vi "Funnel Edit.vi"() -> ()   [LabVIEW 2016]
uses:
  <userlib>/LevyLab/Relay Box/Type_defs/Resistor--enum.ctl
  Global Variables.vi
panel:
  in  "Set Resistance":T1=enum."1G ohm"
  in  "Index":i32=8
  in  "Direction":u16(ring) items=["Forward", "Backward"]
  in  "Enabled":bool=TRUE
  in  "Voltage Schedule":u16(ring) items=["Constant", "Ramp", "Fn. Generator", "Formula"]
  in  "Apply to All":bool
  in  "Smooth Segments":dbl=12.0
  in  "Speed Schedule":u16(ring) items=["Constant", "Ramp", "Fn. Generator", "Formula"]
  in  "Speed (µm/s)":dbl=8.0 min=1e-09
  in  "Voltage (V)":dbl=8.0
  in  "Speed Settings":bool
  in  "Voltage Settings":bool
  in  "Bottom Segs.":dbl=0.1
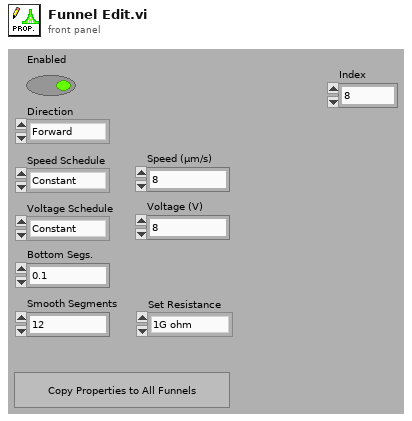
[diagram p1: front panel]
types:
  T1 = typedef "Resistor--enum.ctl" = enum16{"open", "discharge tip", "0 ohms", "100k ohm", "10M ohm", "1G ohm"}
  T2 = enum32{"invalid app kind", "Development System", "Run Time System", "Student Edition", "Embedded LabVIEW", "Evaluation", "Custom"}
  T3 = enum32{"Invalid", "Standard", "Closed", "Hidden", "Minimized", "Maximized"}
  T4 = typedef "Funnel Properties - cluster.ctl" = cluster{"Enabled":bool, "Direction":u16, "Smooth Segments":dbl, "Bottom Segs.":dbl, "Speed (um/s)":T5, "Voltage (V)":T5, "Set Resistance":T1}
  T5 = typedef "Voltage - cluster.ctl" = cluster{"Schedule":T6, "Value":dbl, "Start Value":dbl, "End Value":dbl, "Min Value":dbl, "Max Value":dbl, "Duty Cycle (%)":dbl, "Signal Type":T7, "Cycle Number":dbl, "Phase (degrees)":dbl, "formula":string, "formula length (nm)":dbl, "formula resolution (nm)":dbl}
  T6 = typedef "Schedule - enum.ctl" = enum16{"Constant", "Ramp", "Fn. Generator", "Formula"}
  T7 = typedef "Signal Type - enum.ctl" = enum16{"Sine Wave", "Triangle Wave", "Square Wave", "Sawtooth Wave"}
  T8 = cluster{"Core":cluster{"Current VI Reference":refnum<vi>, "Close Panel on Exit?":bool}}
  T9 = cluster{"Current VI Reference":refnum<vi>, "Close Panel on Exit?":bool}
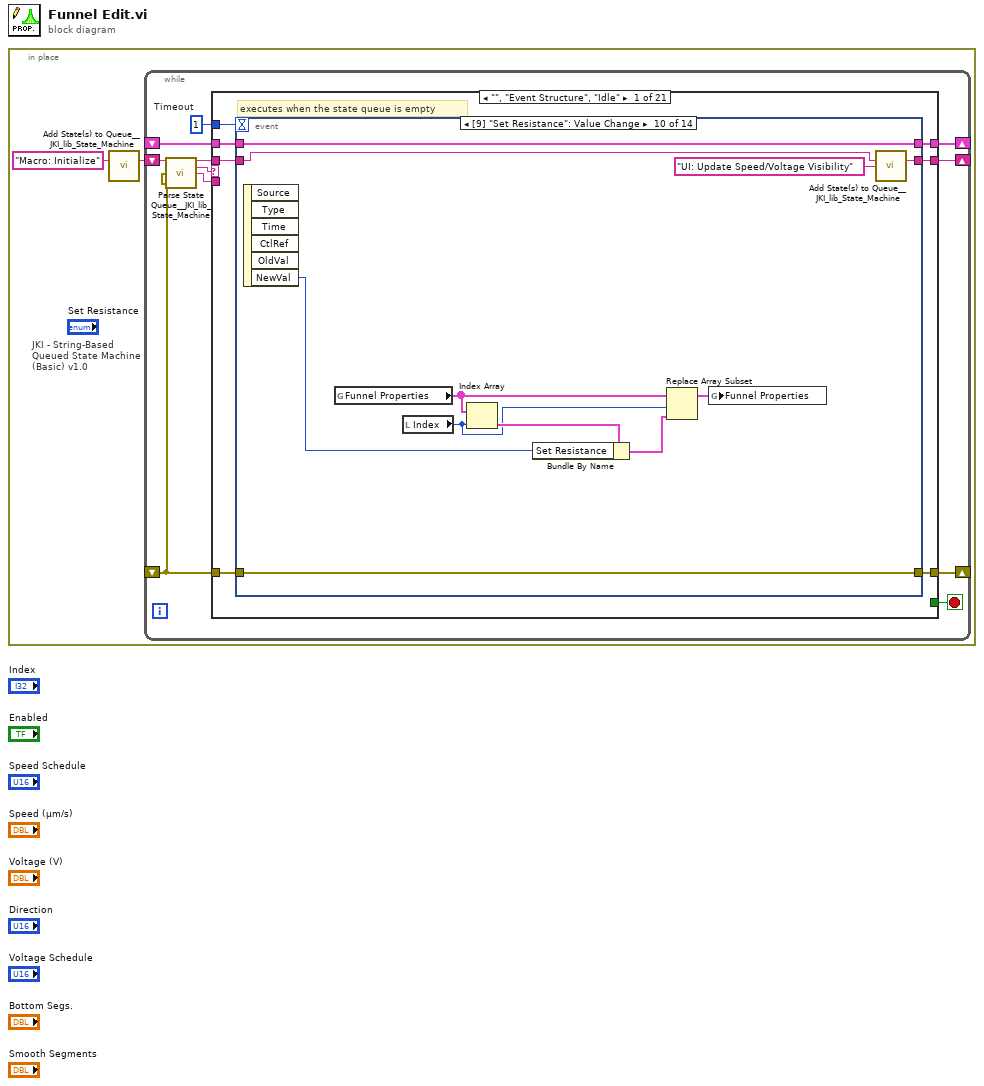
[diagram p0: block diagram]
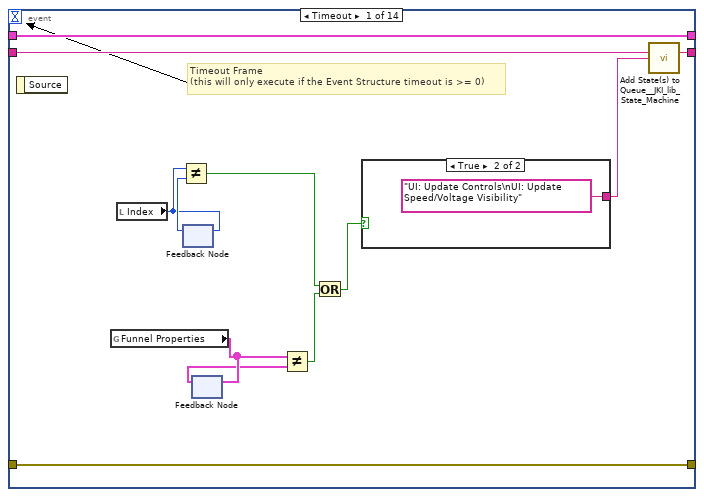
[diagram p2: hidden frame]
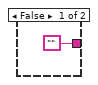
[diagram p3: hidden frame]
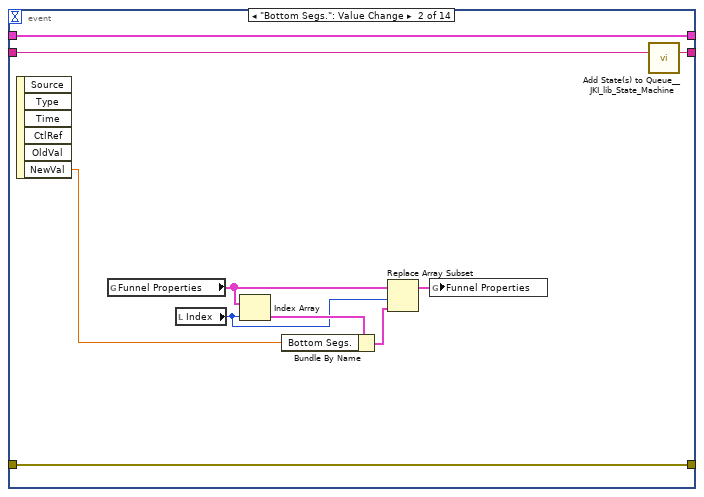
[diagram p4: hidden frame]
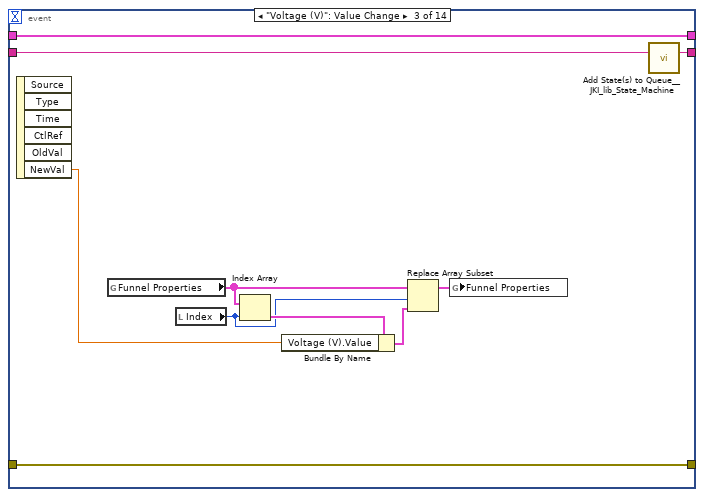
[diagram p5: hidden frame]
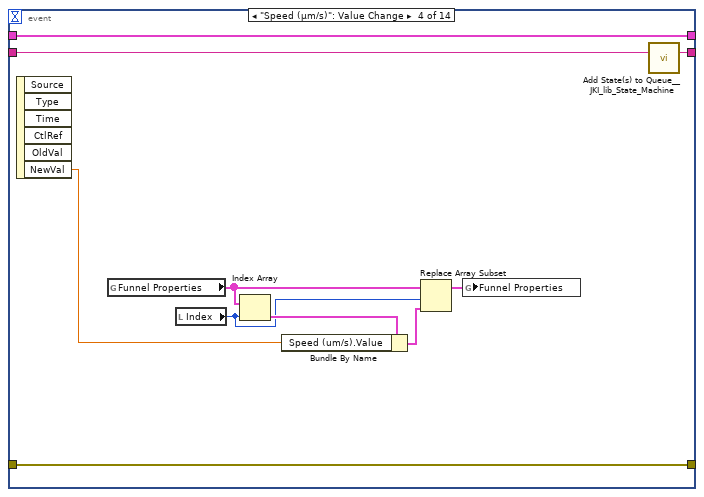
[diagram p6: hidden frame]
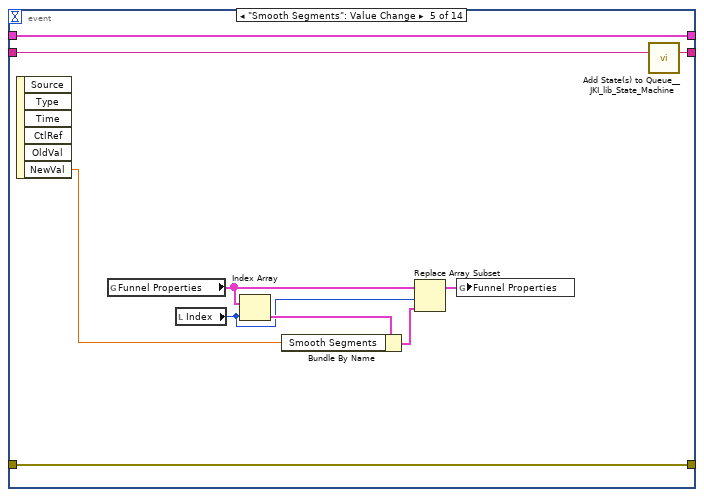
[diagram p7: hidden frame]
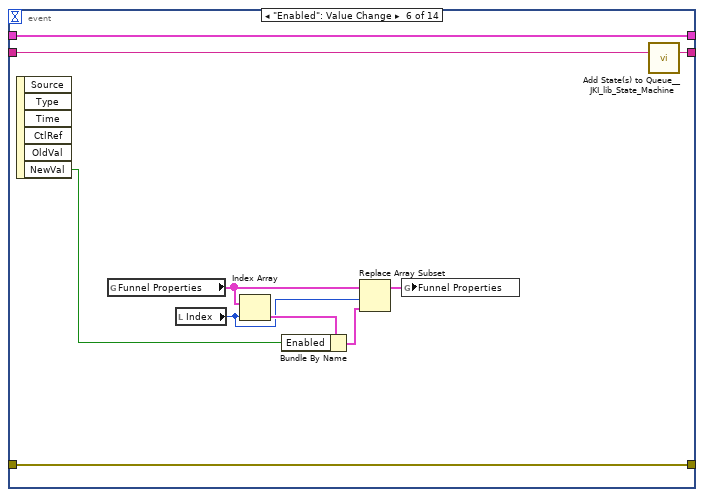
[diagram p8: hidden frame]
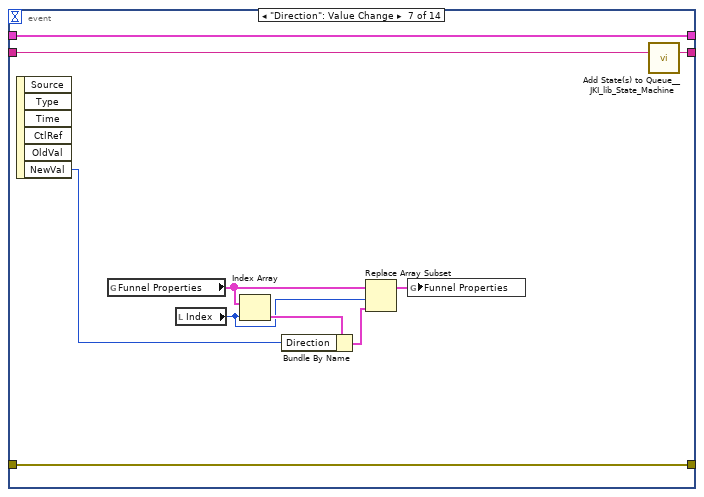
[diagram p9: hidden frame]
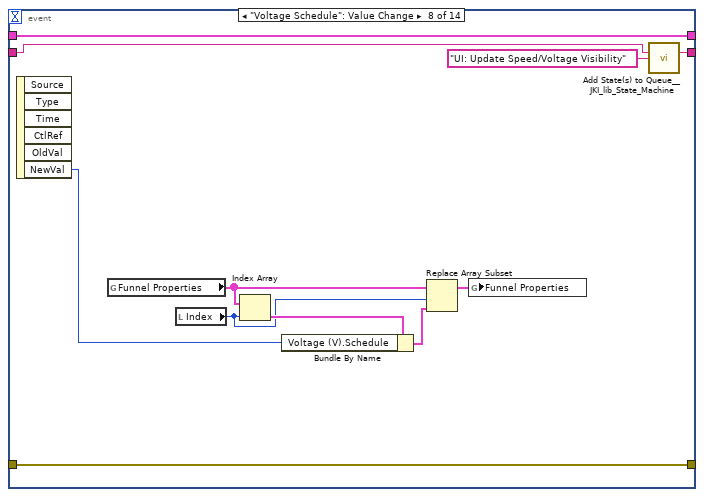
[diagram p10: hidden frame]
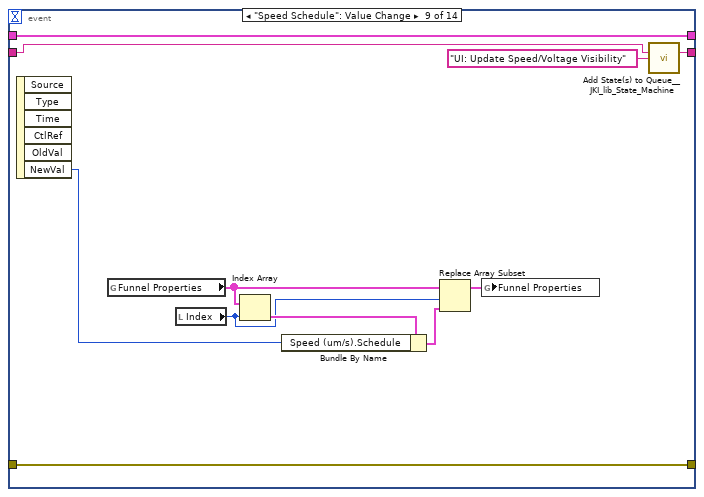
[diagram p11: hidden frame]
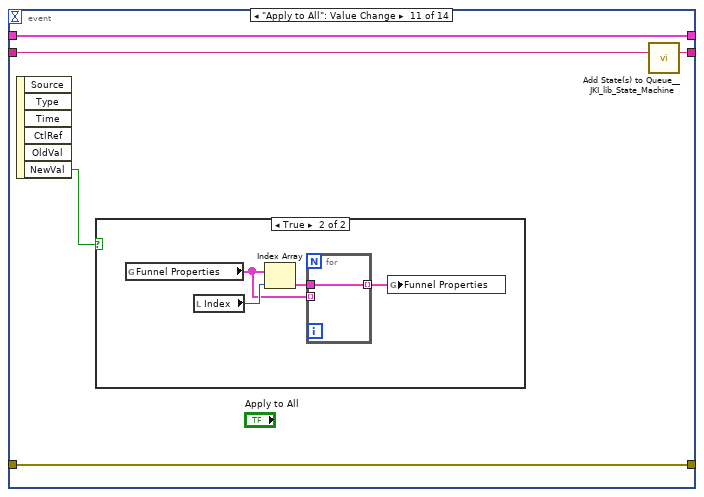
[diagram p12: hidden frame]
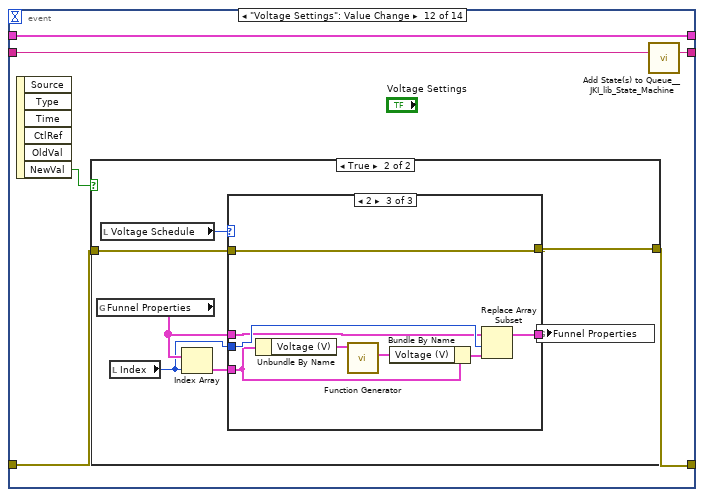
[diagram p14: hidden frame]
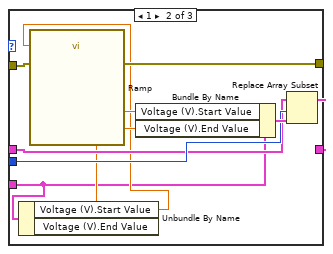
[diagram p17: hidden frame]
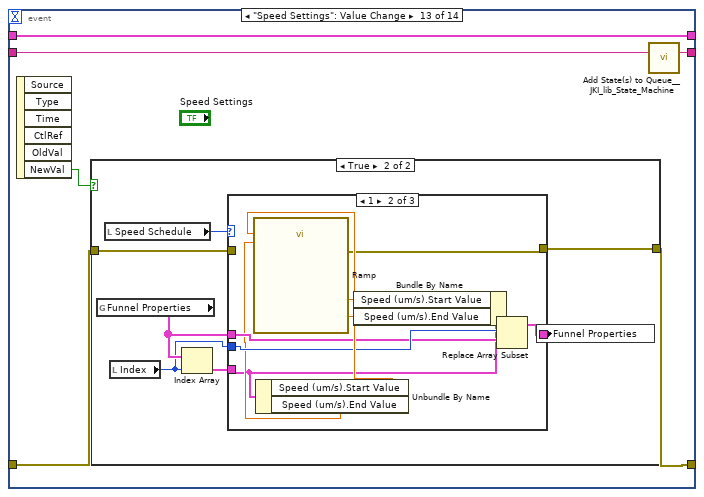
[diagram p18: hidden frame]
diagram:
  n1 = in-place {
    n2 = call <vilib>:"Add State(s) to Queue__JKI_lib_State_Machine.vi"("State(s) in (\"\")"="Macro: Initialize") -> ("States Out"=w2:string)  [unwired: 14 in]
    n3 = while "JKI - String-Based Queued State Machine (Basic) v1.0" {
      shift-right: [w6] -> _
      shift-left: _ -> [w5]
      shift-right: [w9] -> _
      shift-left: _ -> [w3]
      shift-right: [w8] -> _
      shift-left: w2 -> [w10]
      stop <- w7 stop-if-true
      w4 = 1  # Timeout
      n4 = call <vilib>:"Parse State Queue__JKI_lib_State_Machine.vi"("State Queue"=w10, "Error In (no error)"=w3) -> ("Remaining States"=w12:string, "Current State"=w13:string, "Arguments"=w11:string)  [unwired: 11 in]
      n5 = case shown="\"\", \"Event Structure\", \"Idle\"" w13 {
        selector: w13 -> [_ _ w217 _ _ _ _ _ _ _ _ _ _ _ _ _ _ _ _ _ _]
        tunnel: w12 -> [w20 w216 w221 w239 w245 w250 w254 w259 w265 w269 w273 w289 w295 w313 w324 w350 w355 w365 w369 w373 w377]
        tunnel: w11 -> [_ _ _ _ _ _ _ _ _ _ _ _ w290 _ w318 _ _ _ _ _ _]
        tunnel: w5 -> [w18 w213 w219 w235 w242 w248 w251 _ w263 w266 w271 w287 w293 w311 w320 w347 w352 w362 w366 w370 w374]
        tunnel: [w17 w214 w223 w236 errorcluster {"status"=FALSE, "code"=0, "source"=""} ("error out") w247 w252 w255 w261 w267 w270 w276 w291 w300 w321 w348 w353 w363 w367 w371 w375] -> w9
        tunnel: w3 -> [w16 w214 w222 w236 w241 w247 w252 w255 w260 w267 w270 w276 w292 w310 w322 w348 w353 w363 w367 w371 w375]
        tunnel: [w19 w215 w220 w238 w244 w249 w253 w258 w264 w268 w272 w288 w294 w312 w323 w349 w354 w364 w368 w372 w376] -> w8
        tunnel: [_ _ _ _ _ TRUE _ _ _ _ _ _ _ _ _ _ _ _ _ _ _] -> w7
        tunnel: [w15 w213 w219 w237 w242 w248 w251 w257 w263 w266 w271 w287 w293 w311 w320 w347 w352 w362 w366 w370 w374] -> w6
        tunnel: w4 -> [w14 _ _ _ _ _ _ _ _ _ _ _ _ _ _ _ _ _ _ _ _]
        frame "", "Event Structure", "Idle" {
          # "executes when the state queue is empty"
          n6 = event shown="[9] \"Set Resistance\": Value Change" {
            selector: _ -> [_ _ _ _ _ _ _ _ _ _ _ _ _ _]
            dyn-events: _ -> [_ _ _ _ _ _ _ _ _ _ _ _ _ _]
            timeout: w14 -> [_ _ _ _ _ _ _ _ _ _ _ _ _ _]
            tunnel: w20 -> [w32 w44 w54 w64 w74 w84 w94 w105 w116 w127 w132 w143 w178 w212]
            tunnel: [w31 w43 w53 w63 w73 w83 w93 w104 w115 w126 w131 w142 w177 w211] -> w19
            tunnel: w18 -> [w29 w42 w52 w62 w72 w82 w92 w103 w114 w125 w130 w141 w176 w209]
            tunnel: [w30 w36 w46 w56 w66 w76 w86 w97 w108 w119 w129 w139 w174 w210] -> w17
            tunnel: w16 -> [w30 w36 w46 w56 w66 w76 w86 w97 w108 w119 w129 w140 w175 w210]
            tunnel: [w29 w42 w52 w62 w72 w82 w92 w103 w114 w125 w130 w141 w176 w209] -> w15
            event Timeout {
              # "Timeout Frame\n(this will only execute if the Event Structure timeout is >= 0)"
              n7 = event-data() -> ()  [unwired: 1 in, 1 out]
              n8 = global read "Global Variables.vi" "Funnel Properties"() -> (w25:T4[])
              n9 = local read "Index"() -> (w27:i32)
              n10 = feedback #1() -> (w28:i32)  [unwired: 1 in]
              n11 = Not Equal?(x=w27, y=w28) -> (x != y?=w23:bool)
              n12 = feedback-in #1(w27) -> ()
              n13 = feedback #2() -> (w24:T4[])  [unwired: 1 in]
              n14 = feedback-in #2(w25) -> ()
              n15 = Not Equal?(x=w25, y=w24) -> (x != y?=w22:bool)
              n16 = Or(x=w23, y=w22) -> (x .or. y?=w21:bool)
              n17 = case shown="True" w21 {
                tunnel: ["" "UI: Update Controls\nUI: Update Speed/Voltage Visibility"] -> w26
                frame False {
                }
                frame True {
                }
              }
              n18 = call <vilib>:"Add State(s) to Queue__JKI_lib_State_Machine.vi"("State(s) in (\"\")"=w32, "State(s) at Back (\"\")"=w26) -> ("States Out"=w31:string)  [unwired: 13 in]
            }
            event "Bottom Segs.": Value Change {
              n19 = event-data() -> ("NewVal"=w40:dbl)  [unwired: 1 in, 5 out]
              n20 = global read "Global Variables.vi" "Funnel Properties"() -> (w38:T4[])
              n21 = local read "Index"() -> (w35:i32)
              n22 = Index Array(array=w38, index=w35) -> (element=w41:T4)
              n23 = Bundle By Name(cluster=w41, "Bottom Segs."=w40) -> (w39:T4)
              n24 = Replace Array Subset(array=w38, new element=w39, index=w35) -> (w37:T4[])
              n25 = global write "Global Variables.vi" "Funnel Properties"(w37) -> ()
              n26 = call <vilib>:"Add State(s) to Queue__JKI_lib_State_Machine.vi"("State(s) in (\"\")"=w44) -> ("States Out"=w43:string)  [unwired: 14 in]
            }
            event "Voltage (V)": Value Change {
              n27 = event-data() -> ("NewVal"=w50:dbl)  [unwired: 1 in, 5 out]
              n28 = global read "Global Variables.vi" "Funnel Properties"() -> (w48:T4[])
              n29 = local read "Index"() -> (w45:i32)
              n30 = Index Array(array=w48, index=w45) -> (element=w51:T4)
              n31 = Bundle By Name(cluster=w51, "Voltage (V).Value"=w50) -> (w49:T4)
              n32 = Replace Array Subset(array=w48, new element=w49, index=w45) -> (w47:T4[])
              n33 = global write "Global Variables.vi" "Funnel Properties"(w47) -> ()
              n34 = call <vilib>:"Add State(s) to Queue__JKI_lib_State_Machine.vi"("State(s) in (\"\")"=w54) -> ("States Out"=w53:string)  [unwired: 14 in]
            }
            event "Speed (µm/s)": Value Change {
              n35 = event-data() -> ("NewVal"=w60:dbl)  [unwired: 1 in, 5 out]
              n36 = global read "Global Variables.vi" "Funnel Properties"() -> (w58:T4[])
              n37 = local read "Index"() -> (w55:i32)
              n38 = Index Array(array=w58, index=w55) -> (element=w61:T4)
              n39 = Bundle By Name(cluster=w61, "Speed (um/s).Value"=w60) -> (w59:T4)
              n40 = Replace Array Subset(array=w58, new element=w59, index=w55) -> (w57:T4[])
              n41 = global write "Global Variables.vi" "Funnel Properties"(w57) -> ()
              n42 = call <vilib>:"Add State(s) to Queue__JKI_lib_State_Machine.vi"("State(s) in (\"\")"=w64) -> ("States Out"=w63:string)  [unwired: 14 in]
            }
            event "Smooth Segments": Value Change {
              n43 = event-data() -> ("NewVal"=w70:dbl)  [unwired: 1 in, 5 out]
              n44 = global read "Global Variables.vi" "Funnel Properties"() -> (w68:T4[])
              n45 = local read "Index"() -> (w65:i32)
              n46 = Index Array(array=w68, index=w65) -> (element=w71:T4)
              n47 = Bundle By Name(cluster=w71, "Smooth Segments"=w70) -> (w69:T4)
              n48 = Replace Array Subset(array=w68, new element=w69, index=w65) -> (w67:T4[])
              n49 = global write "Global Variables.vi" "Funnel Properties"(w67) -> ()
              n50 = call <vilib>:"Add State(s) to Queue__JKI_lib_State_Machine.vi"("State(s) in (\"\")"=w74) -> ("States Out"=w73:string)  [unwired: 14 in]
            }
            event "Enabled": Value Change {
              n51 = event-data() -> ("NewVal"=w80:bool)  [unwired: 1 in, 5 out]
              n52 = global read "Global Variables.vi" "Funnel Properties"() -> (w78:T4[])
              n53 = local read "Index"() -> (w75:i32)
              n54 = Index Array(array=w78, index=w75) -> (element=w81:T4)
              n55 = Bundle By Name(cluster=w81, "Enabled"=w80) -> (w79:T4)
              n56 = Replace Array Subset(array=w78, new element=w79, index=w75) -> (w77:T4[])
              n57 = global write "Global Variables.vi" "Funnel Properties"(w77) -> ()
              n58 = call <vilib>:"Add State(s) to Queue__JKI_lib_State_Machine.vi"("State(s) in (\"\")"=w84) -> ("States Out"=w83:string)  [unwired: 14 in]
            }
            event "Direction": Value Change {
              n59 = event-data() -> ("NewVal"=w90:u16)  [unwired: 1 in, 5 out]
              n60 = global read "Global Variables.vi" "Funnel Properties"() -> (w88:T4[])
              n61 = local read "Index"() -> (w85:i32)
              n62 = Index Array(array=w88, index=w85) -> (element=w91:T4)
              n63 = Bundle By Name(cluster=w91, "Direction"=w90) -> (w89:T4)
              n64 = Replace Array Subset(array=w88, new element=w89, index=w85) -> (w87:T4[])
              n65 = global write "Global Variables.vi" "Funnel Properties"(w87) -> ()
              n66 = call <vilib>:"Add State(s) to Queue__JKI_lib_State_Machine.vi"("State(s) in (\"\")"=w94) -> ("States Out"=w93:string)  [unwired: 14 in]
            }
            event "Voltage Schedule": Value Change {
              n67 = event-data() -> ("NewVal"=w101:u16)  [unwired: 1 in, 5 out]
              n68 = global read "Global Variables.vi" "Funnel Properties"() -> (w99:T4[])
              n69 = local read "Index"() -> (w95:i32)
              n70 = Index Array(array=w99, index=w95) -> (element=w102:T4)
              n71 = Bundle By Name(cluster=w102, "Voltage (V).Schedule"=w101) -> (w100:T4)
              n72 = Replace Array Subset(array=w99, new element=w100, index=w95) -> (w98:T4[])
              n73 = global write "Global Variables.vi" "Funnel Properties"(w98) -> ()
              n74 = call <vilib>:"Add State(s) to Queue__JKI_lib_State_Machine.vi"("State(s) in (\"\")"=w105, "State(s) at Back (\"\")"="UI: Update Speed/Voltage Visibility" ("State(s) at Back (\"\")")) -> ("States Out"=w104:string)  [unwired: 13 in]
            }
            event "Speed Schedule": Value Change {
              n75 = event-data() -> ("NewVal"=w112:u16)  [unwired: 1 in, 5 out]
              n76 = global read "Global Variables.vi" "Funnel Properties"() -> (w110:T4[])
              n77 = local read "Index"() -> (w106:i32)
              n78 = Index Array(array=w110, index=w106) -> (element=w113:T4)
              n79 = Bundle By Name(cluster=w113, "Speed (um/s).Schedule"=w112) -> (w111:T4)
              n80 = Replace Array Subset(array=w110, new element=w111, index=w106) -> (w109:T4[])
              n81 = global write "Global Variables.vi" "Funnel Properties"(w109) -> ()
              n82 = call <vilib>:"Add State(s) to Queue__JKI_lib_State_Machine.vi"("State(s) in (\"\")"=w116, "State(s) at Back (\"\")"="UI: Update Speed/Voltage Visibility" ("State(s) at Back (\"\")")) -> ("States Out"=w115:string)  [unwired: 13 in]
            }
            event Value Change {
              n83 = event-data() -> ("NewVal"=w123:T1)  [unwired: 1 in, 5 out]
              n84 = global read "Global Variables.vi" "Funnel Properties"() -> (w121:T4[])
              n85 = local read "Index"() -> (w117:i32)
              n86 = Index Array(array=w121, index=w117) -> (element=w124:T4)
              n87 = Bundle By Name(cluster=w124, "Set Resistance"=w123) -> (w122:T4)
              n88 = Replace Array Subset(array=w121, new element=w122, index=w117) -> (w120:T4[])
              n89 = global write "Global Variables.vi" "Funnel Properties"(w120) -> ()
              n90 = call <vilib>:"Add State(s) to Queue__JKI_lib_State_Machine.vi"("State(s) in (\"\")"=w127, "State(s) at Back (\"\")"="UI: Update Speed/Voltage Visibility" ("State(s) at Back (\"\")")) -> ("States Out"=w126:string)  [unwired: 13 in]
            }
            event "Apply to All": Value Change {
              n91 = event-data() -> ("NewVal"=w128:bool)  [unwired: 1 in, 5 out]
              n92 = case shown="True" w128 {
                frame False {
                }
                frame True {
                  n93 = global read "Global Variables.vi" "Funnel Properties"() -> (w133:T4[])
                  n94 = local read "Index"() -> (w136:i32)
                  n95 = Index Array(array=w133, index=w136) -> (element=w135:T4)
                  n96 = for {
                    tunnel: w135 -> [w137]
                    tunnel: [w137] -> w134 mode=indexing
                    tunnel: w133 -> [_] mode=indexing
                  }
                  n97 = global write "Global Variables.vi" "Funnel Properties"(w134) -> ()
                }
              }
              n98 = call <vilib>:"Add State(s) to Queue__JKI_lib_State_Machine.vi"("State(s) in (\"\")"=w132) -> ("States Out"=w131:string)  [unwired: 14 in]
            }
            event "Voltage Settings": Value Change {
              n99 = event-data() -> ("NewVal"=w138:bool)  [unwired: 1 in, 5 out]
              n100 = case shown="True" w138 {
                tunnel: w140 -> [w144 w150]
                tunnel: [w144 w149] -> w139
                frame False {
                }
                frame True {
                  n101 = global read "Global Variables.vi" "Funnel Properties"() -> (w146:T4[])
                  n102 = local read "Voltage Schedule"() -> (w151:u16)
                  n103 = local read "Index"() -> (w145:i32)
                  n104 = Index Array(array=w146, index=w145) -> (element=w147:T4)
                  n105 = case shown="2" w151 {
                    tunnel: w150 -> [w153 w164 w168]
                    tunnel: [w153 w157 w168] -> w149
                    tunnel: [w152 w158 w169] -> w148
                    tunnel: w147 -> [_ w154 w167]
                    tunnel: w146 -> [w152 w159 w170]
                    tunnel: w145 -> [_ w160 w171]
                    frame 0, Default {
                    }
                    frame 1 {
                      n106 = Unbundle By Name(w154) -> ("Voltage (V).Start Value"=w156:dbl, "Voltage (V).End Value"=w155:dbl)
                      n107 = call "Ramp.vi"("Start Value"=w156, "End Value"=w155, "error in (no error)"=w164) -> ("End Value"=w162:dbl, "Start Value"=w163:dbl, "error out"=w157:errorcluster)  [unwired: 13 in, 1 out]
                      n108 = Bundle By Name(cluster=w154, "Voltage (V).Start Value"=w163, "Voltage (V).End Value"=w162) -> (w161:T4)
                      n109 = Replace Array Subset(array=w159, new element=w161, index=w160) -> (w158:T4[])
                    }
                    frame 2 {
                      n110 = Unbundle By Name(w167) -> ("Voltage (V)"=w165:T5)
                      n111 = call "Function Generator.vi"("Properties in"=w165) -> ("Properties out"=w166:T5)  [unwired: 9 in, 1 out]
                      n112 = Bundle By Name(cluster=w167, "Voltage (V)"=w166) -> (w172:T4)
                      n113 = Replace Array Subset(array=w170, new element=w172, index=w171) -> (w169:T4[])
                    }
                  }
                  n114 = global write "Global Variables.vi" "Funnel Properties"(w148) -> ()
                }
              }
              n115 = call <vilib>:"Add State(s) to Queue__JKI_lib_State_Machine.vi"("State(s) in (\"\")"=w143) -> ("States Out"=w142:string)  [unwired: 14 in]
            }
            event "Speed Settings": Value Change {
              n116 = event-data() -> ("NewVal"=w173:bool)  [unwired: 1 in, 5 out]
              n117 = case shown="True" w173 {
                tunnel: w175 -> [w179 w185]
                tunnel: [w179 w184] -> w174
                frame False {
                }
                frame True {
                  n118 = global read "Global Variables.vi" "Funnel Properties"() -> (w181:T4[])
                  n119 = local read "Speed Schedule"() -> (w186:u16)
                  n120 = local read "Index"() -> (w180:i32)
                  n121 = Index Array(array=w181, index=w180) -> (element=w182:T4)
                  n122 = case shown="1" w186 {
                    tunnel: w185 -> [w188 _ w202]
                    tunnel: [w188 w194 w202] -> w184
                    tunnel: [w187 w193 w203] -> w183
                    tunnel: w182 -> [_ w189 w201]
                    tunnel: w181 -> [w187 w191 w204]
                    tunnel: w180 -> [_ w192 w205]
                    frame 0, Default {
                    }
                    frame 1 {
                      n123 = Unbundle By Name(w189) -> ("Speed (um/s).Start Value"=w195:dbl, "Speed (um/s).End Value"=w190:dbl)
                      n124 = call "Ramp.vi"("Start Value"=w195, "End Value"=w190) -> ("End Value"=w197:dbl, "Start Value"=w198:dbl, "error out"=w194:errorcluster)  [unwired: 14 in, 1 out]
                      n125 = Bundle By Name(cluster=w189, "Speed (um/s).Start Value"=w198, "Speed (um/s).End Value"=w197) -> (w196:T4)
                      n126 = Replace Array Subset(array=w191, new element=w196, index=w192) -> (w193:T4[])
                    }
                    frame 2 {
                      n127 = Unbundle By Name(w201) -> ("Speed (um/s)"=w199:T5)
                      n128 = call "Function Generator.vi"("Properties in"=w199) -> ("Properties out"=w200:T5)  [unwired: 9 in, 1 out]
                      n129 = Bundle By Name(cluster=w201, "Speed (um/s)"=w200) -> (w206:T4)
                      n130 = Replace Array Subset(array=w204, new element=w206, index=w205) -> (w203:T4[])
                    }
                  }
                  n131 = global write "Global Variables.vi" "Funnel Properties"(w183) -> ()
                }
              }
              n132 = call <vilib>:"Add State(s) to Queue__JKI_lib_State_Machine.vi"("State(s) in (\"\")"=w178) -> ("States Out"=w177:string)  [unwired: 14 in]
            }
            event Panel Close? {
              # "Discard the event because we'll close the front panel ourselves in Macro: Exit"
              # "Close Panel button (pressed) Event\n(this executes Macro: Exit to terminate the VI)"
              n133 = event-data() -> ()  [unwired: 1 in, 1 out]
              n134 = event-data("Discard?"=TRUE) -> ()  [unwired: 1 in, 1 out]
              n135 = call <vilib>:"Add State(s) to Queue__JKI_lib_State_Machine.vi"("State(s) in Front (\"\")"="Macro: Exit", "State(s) in (\"\")"=w212) -> ("States Out"=w211:string)  [unwired: 13 in]
            }
          }
        }
        frame "---------- Core ----------" {
          # "Do not put any code in this frame.\n(it is a separator no-op)"
          n136 = call <vilib>:"Add State(s) to Queue__JKI_lib_State_Machine.vi"("State(s) in (\"\")"=w216) -> ("States Out"=w215:string)  [unwired: 14 in]
        }
        frame Default {
          w226 = 42 items=["No error", "Argument error", "Memory is full", "Out of zone", "End of file", "File already open", "Generic file I/O error", "File not found", "File permission error", "Disk is full", "Duplicate path", "Too many files open", "System feature not enabled", "Resource file not found", "Cannot add resource", "Resource not found", "Image not found", "Image memory error", "Pen does not exist", "Config type invalid", "Config token not found", "Config parse error", "Config memory error", "Bad external code format", "Bad external code offset", "External code not present", "Null window", "Destroy window error", "Null menu", "Print aborted", "Bad print record", "Print driver error", "Windows error during printing", "Memory error during printing", "Print dialog error", "Generic print error", "Invalid device refnum", "Device not found", "Device parameter error", "Device unit error", "Cannot open device", "Device call aborted", "Generic error", "Cancelled by user", "Object ID too low", "Object ID too high", "Object not in heap", "Unknown heap", "Unknown object (invalid DefProc)", "Unknown object (DefProc not in table)", "Message out of range", "Invalid (null) method", "Unknown message", "Manager call not supported", "Bad address", "Network operation in progress", "Network operation timed out", "Connection is busy", "Network attribute not supported", "Network error", "Address in use", "System out of memory", "Connection aborted", "Connection refused", "Not connected", "Already connected", "Connection closed", "Initialization error (interapplication manager)", "Bad occurrence", "Wait on unbound occurrence handler", "Occurrence queue overflow", "Datalog type conflict", "Unused", "Unrecognized type (interapplication manager)", "Memory corrupt", "Failed to make temporary DLL", "Old CIN version", "Drag socket not found", "Failed to load drop-object", "Failed to register OLE object", "Failed to release OLE object", "Format specifier type mismatch", "Unknown format specifier", "Too few format specifiers", "Too many format specifiers", "Scan failed", "Newer CIN version", "Error converting to variant", "Runtime menu error", "Password tampered", "Variant attribute not found", "Incompatible variant data type", "Event data is not available", "Event Store is not present", "Occurrence is not found", "Event Queue is not created", "Event info is not available", "Refnum passed is NULL", "Error retrieving Class GUID", "Error retrieving CoClass GUID", "Error retrieving TypeLib GUID.", "Bad built application magic bytes.", "Specific driver is different from the specific driver associated with the Logical Name.", "There is no session opened to the class driver.", "Max Error", "MAX - Error with config objects", "MAX - Error loading configuration", "MAX - Group not supported"]
          # "Current State"
          # "Do not delete, rename, or modify this frame.\n(this is used to capture unhandled states and typos)"
          # "Handle mistyped state name (developer tool)"
          n137 = Format Into String(format string="Software Exception: Unhandled State \"%s\"." ("message"), error in=w222, w217) -> (resulting string=w225:string, error out=w224:errorcluster)  [unwired: 1 in]
          n138 = call <vilib>:"Error Cluster From Error Code.vi"("show call chain? (False)"=TRUE, "error in (no error)"=w224, "error message (\"\")"=w225, "error code (0)"=w226) -> ("error out"=w223:errorcluster)  [unwired: 5 in]
          n139 = call <vilib>:"Add State(s) to Queue__JKI_lib_State_Machine.vi"("State(s) in (\"\")"=w221) -> ("States Out"=w220:string)  [unwired: 14 in]
        }
        frame "Initialize Core Data" {
          # "exe?"
          # "If panel starts closed or is an EXE, then close it when we exit"
          # "Do not delete, rename, or modify this frame.\n(this is used to determine panel behavior on exit)"
          n140 = property class="VI"() -> ("Front Panel.Open"=w233:bool)  [unwired: 2 in, 2 out]
          n141 = property class="App"() -> ("App.Kind"=w232:T2)  [unwired: 2 in, 2 out]
          n142 = control-ref of="Current VI Reference"() -> (w234:refnum<vi>)
          n143 = Not(x=w233) -> (.not. x?=w230:bool)
          n144 = Equal?(x=w232, y=T2."Run Time System" ("Application:Kind")) -> (x = y?=w229:bool)
          n145 = Or(x=w230, y=w229) -> (x .or. y?=w228:bool)
          n146 = Bundle By Name(cluster=w235, "Core.Current VI Reference"=w234, "Core.Close Panel on Exit?"=w228) -> (w237:T8)
          n147 = call <vilib>:"Add State(s) to Queue__JKI_lib_State_Machine.vi"("State(s) in (\"\")"=w239) -> ("States Out"=w238:string)  [unwired: 14 in]
        }
        frame "Error Handler" {
          # "Unhandled Error -- Display it"
          # "Handle any errors here.\nYou can also output any states to clean-up after errors occur"
          # "Clear error"
          n148 = call <vilib>:"General Error Handler.vi"("error in (no error)"=w241) -> ()  [unwired: 10 in, 5 out]
          n149 = call <vilib>:"Add State(s) to Queue__JKI_lib_State_Machine.vi"("State(s) in Front (\"\")"="/* Post Error States", "State(s) in (\"\")"=w245) -> ("States Out"=w244:string)  [unwired: 13 in]
        }
        frame "Exit" {
          # "Do not put any code in this frame.\n(No errors that occur here will be handled.)"
          n150 = call <vilib>:"Add State(s) to Queue__JKI_lib_State_Machine.vi"("State(s) in (\"\")"=w250) -> ("States Out"=w249:string)  [unwired: 14 in]
        }
        frame "---------- Data ----------" {
          # "Do not put any code in this frame.\n(It is a separator no-op. You can make a copy of this frame to create a new Data frame)"
          n151 = call <vilib>:"Add State(s) to Queue__JKI_lib_State_Machine.vi"("State(s) in (\"\")"=w254) -> ("States Out"=w253:string)  [unwired: 14 in]
        }
        frame "Data: Initialize" {
          w256 = T9 {"Current VI Reference"=refnum, "Close Panel on Exit?"=FALSE}  # Core
          # "Initialize the shift-register data, here.\n(data names are defined by what you wire into the bundle function)"
          n152 = Bundle("Core"=w256) -> (w257:T8)  [unwired: 1 in]
          n153 = call <vilib>:"Add State(s) to Queue__JKI_lib_State_Machine.vi"("State(s) in (\"\")"=w259) -> ("States Out"=w258:string)  [unwired: 14 in]
        }
        frame "Data: Cleanup" {
          # "Cleanup any data and references, here.\n(this is called automatically, by the Macro: Exit)"
          n154 = Unbundle By Name(w263) -> ("Core.Current VI Reference"=w262:refnum<vi>)
          n155 = Close Reference(reference=w262, error in (no error)=w260) -> (error out=w261:errorcluster)
          n156 = call <vilib>:"Add State(s) to Queue__JKI_lib_State_Machine.vi"("State(s) in (\"\")"=w265) -> ("States Out"=w264:string)  [unwired: 14 in]
        }
        frame "---------- UI ----------" {
          # "Do not put any code in this frame.\n(It is a separator no-op. You can make a copy of this frame to create a new UI frame)"
          n157 = call <vilib>:"Add State(s) to Queue__JKI_lib_State_Machine.vi"("State(s) in (\"\")"=w269) -> ("States Out"=w268:string)  [unwired: 14 in]
        }
        frame "UI: Initialize" {
          # "Initialize the User Interface, here.\n(this is called automatically, by the Macro: Init)"
          n158 = call <vilib>:"Add State(s) to Queue__JKI_lib_State_Machine.vi"("State(s) in (\"\")"=w273) -> ("States Out"=w272:string)  [unwired: 14 in]
        }
        frame "UI: Update Controls" {
          n159 = global read "Global Variables.vi" "Funnel Properties"() -> (w275:T4[])
          n160 = local read "Index"() -> (w280:i32)
          n161 = Index Array(array=w275, index=w280) -> (element=w279:T4)
          n162 = Unbundle By Name(w279) -> ("Enabled"=w281:bool, "Direction"=w282:u16, "Smooth Segments"=w283:dbl, "Bottom Segs."=w284:dbl, "Speed (um/s).Schedule"=w278:T6, "Speed (um/s).Value"=w285:dbl, "Voltage (V).Schedule"=w277:T6, "Voltage (V).Value"=w286:dbl, "Set Resistance"=w274:T1)
          n163 = local write "Enabled"(w281) -> ()
          n164 = local write "Direction"(w282) -> ()
          n165 = local write "Smooth Segments"(w283) -> ()
          n166 = local write "Bottom Segs."(w284) -> ()
          n167 = local write "Speed Schedule"(w278) -> ()
          n168 = local write "Speed (µm/s)"(w285) -> ()
          n169 = local write "Voltage Schedule"(w277) -> ()
          n170 = local write "Voltage (V)"(w286) -> ()
          n171 = local write "Voltage Schedule"(w274) -> ()
          n172 = call <vilib>:"Add State(s) to Queue__JKI_lib_State_Machine.vi"("State(s) in (\"\")"=w289) -> ("States Out"=w288:string)  [unwired: 14 in]
        }
        frame "UI: Cursor Set" {
          # "Argument"
          # "Set and Unset Cursor Busy.\n(Usage: \"UI: Cursor Set >> Busy|Idle\")"
          n173 = case shown="\"Idle\", Default" w290 {
            tunnel: w292 -> [w297 w299]
            tunnel: [w296 w298] -> w291
            frame "Idle", Default {
              n174 = call <vilib>:"Unset Busy.vi"("error in (no error)"=w297) -> ("error out"=w296:errorcluster)  [unwired: 10 in]
            }
            frame "Busy" {
              n175 = call <vilib>:"Set Busy.vi"("error in (no error)"=w299) -> ("error out"=w298:errorcluster)  [unwired: 9 in, 1 out]
            }
          }
          n176 = call <vilib>:"Add State(s) to Queue__JKI_lib_State_Machine.vi"("State(s) in (\"\")"=w295) -> ("States Out"=w294:string)  [unwired: 14 in]
        }
        frame "UI: Update Speed/Voltage Visibility" {
          n177 = local read "Voltage Schedule"() -> (w309:u16)
          n178 = case shown="0" w309 {
            tunnel: [TRUE FALSE] -> w305
            frame 0 {
            }
            frame 1, Default {
            }
          }
          n179 = local read "Speed Schedule"() -> (w308:u16)
          n180 = property on="Voltage (V)" class="DigNum (strict)"(error in=w310, "Visible"=w305) -> (error out=w306:errorcluster)  [unwired: 1 in, 1 out]
          n181 = case shown="0" w308 {
            tunnel: [TRUE FALSE] -> w301
            frame 0 {
            }
            frame 1, Default {
            }
          }
          n182 = Not(x=w305) -> (.not. x?=w304:bool)
          n183 = property on="Voltage Settings" class="Bool"(error in=w306, "Visible"=w304) -> (error out=w303:errorcluster)  [unwired: 1 in, 1 out]
          n184 = property on="Speed (µm/s)" class="DigNum (strict)"(error in=w303, "Visible"=w301) -> (error out=w302:errorcluster)  [unwired: 1 in, 1 out]
          n185 = Not(x=w301) -> (.not. x?=w307:bool)
          n186 = property on="Speed Settings" class="Bool"(error in=w302, "Visible"=w307) -> (error out=w300:errorcluster)  [unwired: 1 in, 1 out]
          n187 = call <vilib>:"Add State(s) to Queue__JKI_lib_State_Machine.vi"("State(s) in (\"\")"=w313) -> ("States Out"=w312:string)  [unwired: 14 in]
        }
        frame "UI: Front Panel State" {
          # "Argument"
          # "Set Front Panel Open or Closed\n(Usage: \"UI: Front Panel State >> Open|Close\")"
          n188 = Unbundle By Name(w320) -> ("Core.Current VI Reference"=w319:refnum<vi>)
          n189 = case shown="\"Open\", Default" w318 {
            tunnel: w322 -> [w328 w341]
            tunnel: [w330 w342] -> w321
            tunnel: w319 -> [w329 w339]
            frame "Open", Default {
              n190 = property class="VI"(reference=w329, error in=w328) -> (reference out=w326:refnum<vi>, error out=w327:errorcluster, "Front Panel.Open"=w325:bool)
              n191 = case shown="False" w325 {
                tunnel: [w333 w336] -> w330
                tunnel: w327 -> [w332 w336]
                tunnel: w326 -> [w331 _]
                frame False {
                  n192 = invoke class="VI" method="FP.Open"(reference=w331, error in=w332, "Activate"=TRUE, "State"=T3."Standard") -> (error out=w333:errorcluster)  [unwired: 1 in, 4 out]
                }
                frame True {
                }
              }
            }
            frame "Close" {
              n193 = property class="VI"(reference=w339, error in=w341) -> (reference out=w338:refnum<vi>, error out=w340:errorcluster, "Front Panel.Open"=w337:bool)
              n194 = case shown="True" w337 {
                tunnel: [w343 w346] -> w342
                tunnel: w340 -> [w343 w345]
                tunnel: w338 -> [_ w344]
                frame False {
                }
                frame True {
                  n195 = invoke class="VI" method="FP.Close"(reference=w344, error in=w345) -> (error out=w346:errorcluster)  [unwired: 1 in, 2 out]
                }
              }
            }
          }
          n196 = call <vilib>:"Add State(s) to Queue__JKI_lib_State_Machine.vi"("State(s) in (\"\")"=w324) -> ("States Out"=w323:string)  [unwired: 14 in]
        }
        frame "---------- Macro ----------" {
          # "Do not put any code in this frame.\n(It is a separator no-op. You can make a copy of this frame to create a new Macro frame)"
          n197 = call <vilib>:"Add State(s) to Queue__JKI_lib_State_Machine.vi"("State(s) in (\"\")"=w350) -> ("States Out"=w349:string)  [unwired: 14 in]
        }
        frame "Macro: Initialize" {
          w351 = "Data: Initialize\nInitialize Core Data\nUI: Initialize\nUI: Update Controls\nUI: Update Speed/Voltage Visibility\nUI: Front Panel State >> Close"  # Data: Initialize Initialize Core Data UI: Initialize UI: Update Controls UI: Update Speed/Voltage Visibility UI: Front Panel State >> Close
          # "Initialization Macro\n(This is called once, when the VI starts)"
          n198 = call <vilib>:"Add State(s) to Queue__JKI_lib_State_Machine.vi"("State(s) in Front (\"\")"=w351, "State(s) in (\"\")"=w355) -> ("States Out"=w354:string)  [unwired: 13 in]
        }
        frame "Macro: Exit" {
          # "Exit Macro\n(This is called once, when the VI exits)"
          n199 = Unbundle By Name(w362) -> ("Core.Close Panel on Exit?"=w361:bool)
          n200 = Select(t="UI: Front Panel State >> Close", s=w361, f="") -> (s? t:f=w358:string)
          n201 = call <vilib>:"Add State(s) to Queue__JKI_lib_State_Machine.vi"("State(s) in (\"\")"=w358, "State(s) at Back (\"\")"="Data: Cleanup\nExit") -> ("States Out"=w356:string)  [unwired: 13 in]
          n202 = call <vilib>:"Add State(s) to Queue__JKI_lib_State_Machine.vi"("State(s) in Front (\"\")"=w356, "State(s) in (\"\")"=w365) -> ("States Out"=w364:string)  [unwired: 13 in]
        }
        frame "---------- New Category ----------" {
          # "Template Separator\n(You can make a copy of, or modify, this frame)"
          n203 = call <vilib>:"Add State(s) to Queue__JKI_lib_State_Machine.vi"("State(s) in (\"\")"=w369) -> ("States Out"=w368:string)  [unwired: 14 in]
        }
        frame "New Category: 1" {
          # "Your code here.\n(You can make a copy of, or modify, this frame)"
          n204 = call <vilib>:"Add State(s) to Queue__JKI_lib_State_Machine.vi"("State(s) in (\"\")"=w373) -> ("States Out"=w372:string)  [unwired: 14 in]
        }
        frame "New Category: 2" {
          # "Your code here.\n(You can make a copy of, or modify, this frame)"
          n205 = call <vilib>:"Add State(s) to Queue__JKI_lib_State_Machine.vi"("State(s) in (\"\")"=w377) -> ("States Out"=w376:string)  [unwired: 14 in]
        }
      }
    }
  }
